vi "InitPressureAndTimeSamples.vi"   [LabVIEW 2013]
uses:
  GlobalVariables/PressureAndTimeSamples.vi
types:
  T1 = cluster{"TimeSamples":dbl[], "PressureSamples":dbl[]}
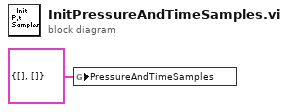
[diagram p0: block diagram]
diagram:
  n1 = global write "PressureAndTimeSamples.vi" "PressureAndTimeSamples"(T1 {"TimeSamples"=[], "PressureSamples"=[]} ("PressureAndTimeSamples")) -> ()
